vi "Read (Measurements).vi"(0 "VISA resource name":refnum<visa-resource-name>, 5 "Timeout (10000 ms)":i32=10000 format="%#.6g", 11 "error in (no error)":errorcluster) -> (3 "Voltage Measurements":sgl[](array[numeric]), 4 "VISA resource name out":refnum<visa-resource-name>, 6 "Current Measurements":sgl[](array[numeric]), 8 "Resistance Measurements":sgl[](array[numeric]), 10 "Timestamp Measurements":sgl[](array[numeric]), 14 "Status Byte":sgl[](array[numeric]), 15 "error out":errorcluster)   [LabVIEW 2022 SP3, in "Keithley 24XX.lvlib"]
doc: "Reads data for voltage, current, resistance, timestamp, and status. These readings are then provided in separate arrays for each type of reading."
uses:
  <instrlib>/Keithley 24XX/Keithley 24XX.lvlib
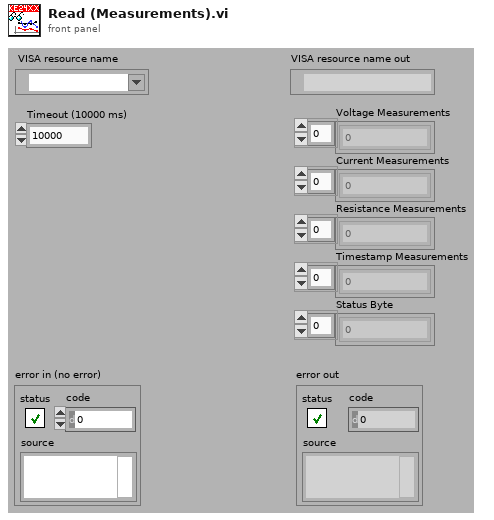
[diagram p1: front panel]
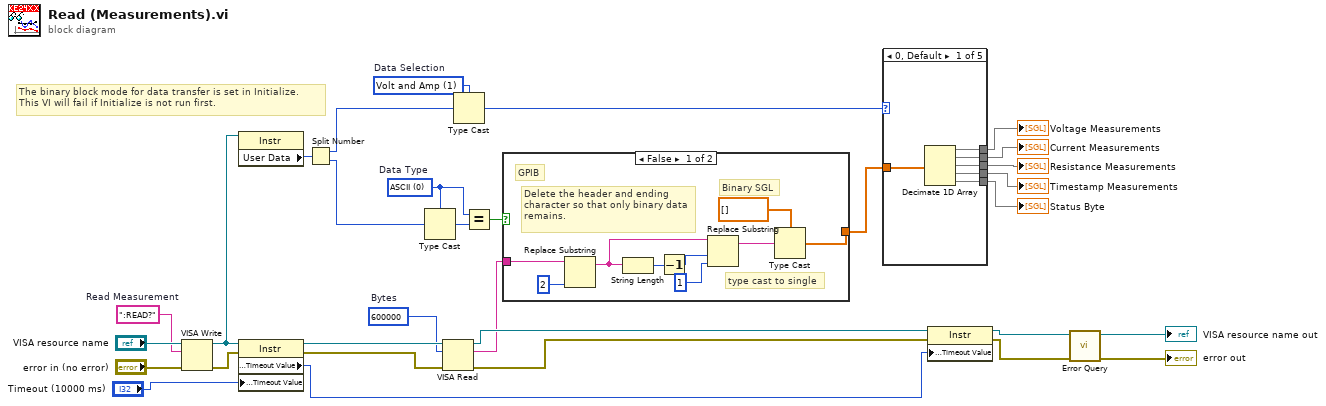
[diagram p0: block diagram]
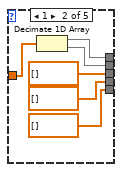
[diagram p2: hidden frame]
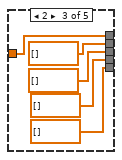
[diagram p3: hidden frame]
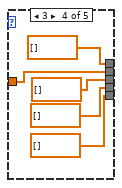
[diagram p4: hidden frame]
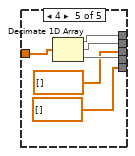
[diagram p5: hidden frame]
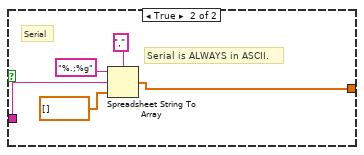
[diagram p6: hidden frame]
diagram:
  w12 = u16 1 items=["All", "Volt and Amp", "Volt", "Amp"]  # Data Selection
  w15 = u16 0 items=["ASCII", "Binary (Single Precision Real)"]  # Data Type
  w29 = ":READ?"  # Read Measurement
  w21 = u32 600000  # Bytes
  # "The binary block mode for data transfer is set in Initialize.  \nThis VI will fail if Initialize is not run first."
  n1 = VISA Write(VISA resource name="VISA resource name", write buffer=w29, error in (no error)="error in (no error)") -> (VISA resource name out=w14:refnum<visa-resource-name>, error out=w28:errorcluster)  [unwired: 1 out]
  n2 = property class="Instr"(reference=w14) -> ("User Data"=w18:u32)  [unwired: 2 in, 1 out]
  n3 = property class="Instr"(reference=w14, error in=w28, "General Settings:Timeout Value"="Timeout (10000 ms)") -> (reference out=w27:refnum<visa-resource-name>, error out=w26:errorcluster, "General Settings:Timeout Value"=w22:u32)
  n4 = Split Number(x=w18) -> (hi(x)=w13:u16, lo(x)=w17:u16)
  n5 = Type Cast(type=w15, x=w17) -> (*(type *) &x=w16:u16)
  n6 = VISA Read(VISA resource name=w27, byte count=w21, error in (no error)=w26) -> (VISA resource name out=w24:refnum<visa-resource-name>, read buffer=w20:string, error out=w23:errorcluster)  [unwired: 1 out]
  n7 = Type Cast(type=w12, x=w13) -> (*(type *) &x=w10:u16)
  n8 = Equal?(x=w15, y=w16) -> (x = y?=w11:bool)
  n9 = case shown="False" w11 {
    tunnel: w20 -> [w40 w45]
    tunnel: [w32 w41] -> w19
    frame False {
      # "Binary SGL"
      # "Delete the header and ending character so that only binary data remains."
      # "GPIB"
      # "type cast to single"
      n10 = Replace Substring(2:2 ("length (len. of substring)"), 5:w40) -> (1:w38:string)  [unwired: 2 in, 1 out]
      n11 = String Length(string=w38) -> (length=w37:i32)
      n12 = Decrement(x=w37) -> (x-1=w36:i32)
      n13 = Replace Substring(2:1 ("length (len. of substring)"), 3:w36, 5:w38) -> (1:w34:string)  [unwired: 1 in, 1 out]
      n14 = Type Cast(type=sgl[] [], x=w34) -> (*(type *) &x=w32:sgl[])
    }
    frame True {
      # "Serial is ALWAYS in ASCII."
      # "Serial"
      n15 = Spreadsheet String To Array(delimiter (Tab)=",", format string="%.;%g", spreadsheet string=w45, array type (2D Dbl)=sgl[] []) -> (array=w41:sgl[])
    }
  }
  n16 = case shown="0, Default" w10 {
    tunnel: w19 -> [w51 w57 w62 w67 w73]
    tunnel: [w50 w56 w62 sgl[] [] w72] -> w9
    tunnel: [w49 w55 sgl[] [] w67 w71] -> w8
    tunnel: [w48 sgl[] [] sgl[] [] sgl[] [] sgl[] []] -> w7
    tunnel: [w47 sgl[] [] sgl[] [] sgl[] [] w70] -> w6
    tunnel: [w46 sgl[] [] sgl[] [] sgl[] [] sgl[] []] -> w5
    frame 0, Default {
      n17 = Decimate 1D Array(w51) -> (w50:sgl[], w49:sgl[], w48:sgl[], w47:sgl[], w46:sgl[])
    }
    frame 1 {
      n18 = Decimate 1D Array(w57) -> (w56:sgl[], w55:sgl[])
    }
    frame 2 {
    }
    frame 3 {
    }
    frame 4 {
      n19 = Decimate 1D Array(w73) -> (w72:sgl[], w71:sgl[], w70:sgl[])
    }
  }
  "Voltage Measurements" <- w9
  "Current Measurements" <- w8
  "Resistance Measurements" <- w7
  "Timestamp Measurements" <- w6
  "Status Byte" <- w5
  n20 = property class="Instr"(reference=w24, error in=w23, "General Settings:Timeout Value"=w22) -> (reference out=w4:refnum<visa-resource-name>, error out=w2:errorcluster)
  n21 = call <instrlib>:"Error Query.vi"("error in (no error)"=w2, "VISA resource name"=w4) -> ("error out"=→"error out":errorcluster, "VISA resource name out"=→"VISA resource name out":refnum<visa-resource-name>)  [unwired: 6 in, 2 out]
